vi "Keithley6221_DeltaRead.vi"(7 "error in (no error)":errorcluster, 8 "memory of # of pts in buffer":i32, 10 "GPIB ADR":u16) -> (0 "error out":errorcluster, 1 "memory of # of pts in buffer update":i32, 2 "Reading":dbl, 3 "Delta Current High":dbl)   [LabVIEW 2012]
panel:
  out "VISA Refnum out":refnum<visa-resource-name>
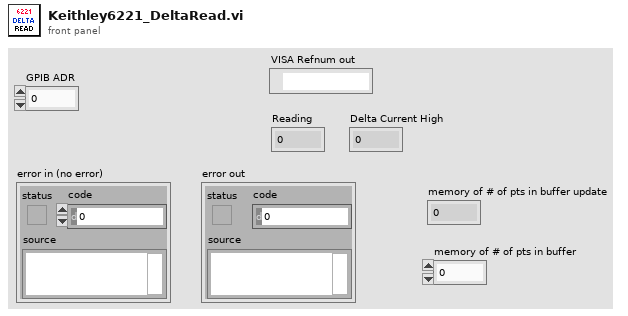
[diagram p1: front panel]
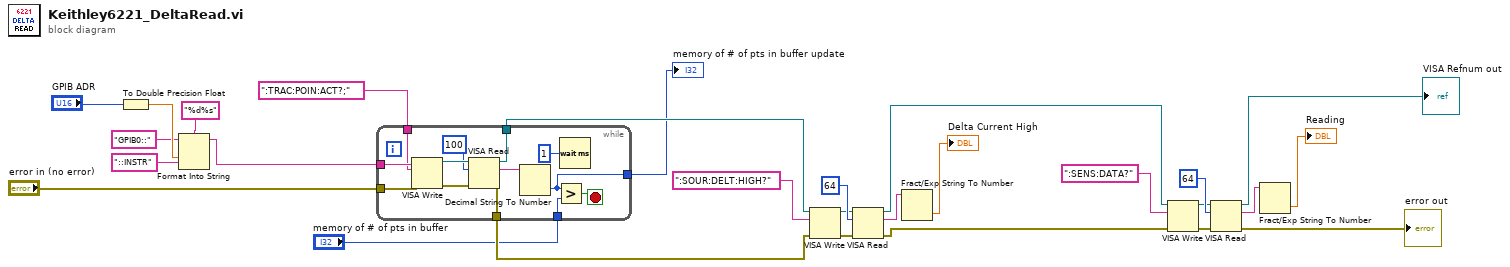
[diagram p0: block diagram]
diagram:
  n1 = To Double Precision Float(number="GPIB ADR") -> (double precision float=w19:dbl)
  n2 = Format Into String(format string="%d%s" ("Removes all labels from the string"), initial string="GPIB0::", w19, "::INSTR") -> (resulting string=w14:string)  [unwired: 1 in, 1 out]
  n3 = while {
    tunnel: w14 -> [w41]
    tunnel: "error in (no error)" -> [w40]
    tunnel: ":TRAC:POIN:ACT?;" ("write buffer") -> [w39]
    tunnel: [w33] -> w4
    tunnel: [w30] -> w1
    tunnel: [w31] -> w5
    tunnel: "memory of # of pts in buffer" -> [w29]
    stop <- w34 stop-if-true
    n4 = VISA Write(VISA resource name=w41, write buffer=w39, error in (no error)=w40) -> (VISA resource name out=w37:refnum<visa-resource-name>, error out=w38:errorcluster)  [unwired: 1 out]
    n5 = VISA Read(VISA resource name=w37, byte count=u32 100, error in (no error)=w38) -> (VISA resource name out=w31:refnum<visa-resource-name>, read buffer=w35:string, error out=w33:errorcluster)  [unwired: 1 out]
    n6 = Decimal String To Number(string=w35) -> (number=w30:i32)  [unwired: 2 in, 1 out]
    n7 = Greater?(x=w30, y=w29) -> (0:w34:bool)
    n8 = Wait (ms)(milliseconds to wait=u32 1) -> ()  [unwired: 1 out]
  }
  "memory of # of pts in buffer update" <- w1
  n9 = VISA Write(VISA resource name=w5, write buffer=":SOUR:DELT:HIGH?", error in (no error)=w4) -> (VISA resource name out=w8:refnum<visa-resource-name>, error out=w10:errorcluster)  [unwired: 1 out]
  n10 = VISA Read(VISA resource name=w8, byte count=u32 64, error in (no error)=w10) -> (VISA resource name out=w6:refnum<visa-resource-name>, read buffer=w11:string, error out=w3:errorcluster)  [unwired: 1 out]
  n11 = Fract/Exp String To Number(string=w11) -> (number=→"Delta Current High":dbl)  [unwired: 3 in, 1 out]
  n12 = VISA Write(VISA resource name=w6, write buffer=":SENS:DATA?", error in (no error)=w3) -> (VISA resource name out=w22:refnum<visa-resource-name>, error out=w24:errorcluster)  [unwired: 1 out]
  n13 = VISA Read(VISA resource name=w22, byte count=u32 64, error in (no error)=w24) -> (VISA resource name out=→"VISA Refnum out":refnum<visa-resource-name>, read buffer=w27:string, error out=→"error out":errorcluster)  [unwired: 1 out]
  n14 = Fract/Exp String To Number(string=w27) -> (number=→"Reading":dbl)  [unwired: 3 in, 1 out]
